vi "Write Page.vi"(4 "Additional Tags":T3(array[cluster]), 5 "Additional Named Tags":cluster{"name":string, "Variant":variant}[](array[cluster]), 6 "Settings":T4={"zlib compression level"=-1, "Max Strip bytes"=8192, "JPEG Quality (85)"=85}, 7 "Details":T5={"ImageDescription"="", "XResolution"=0.0, "YResolution"=0.0, "ResolutionUnit"=enum."Inch", "PhotometricInterpretation"=0, "Compression"=enum."None", "PageName"="", "DocumentName"=""} {"PhotometricInterpretation" items=["PHOTOMETRIC_MINISWHITE"=0, "PHOTOMETRIC_MINISBLACK"=1, "PHOTOMETRIC_RGB"=2, "PHOTOMETRIC_PALETTE"=3, "PHOTOMETRIC_MASK"=4, "PHOTOMETRIC_SEPARATED"=5, "PHOTOMETRIC_YCBCR"=6, "PHOTOMETRIC_CIELAB"=8, "PHOTOMETRIC_ICCLAB"=9, "PHOTOMETRIC_ITULAB"=10, "PHOTOMETRIC_LOGL"=32844, "PHOTOMETRIC_LOGLUV"=32845, "CFA"=32803, "LinearRaw"=34892, "DEPTH"=51177]}, 8 "error in (no error)":errorcluster, 10 "Image":variant, 11 "TIFF Writer in":refnum<class "TIFF Writer.lvclass">) -> (0 "error out":errorcluster, 3 "TIFF Writer out":refnum<class "TIFF Writer.lvclass">)   [LabVIEW 2020, in "LV Tiff.lvlib" / "TIFF Writer.lvclass"]
uses:
  TIFF Writer.lvclass
  _Helpers/Tiff Page Details.ctl
  _Helpers/Page Writer Settings.ctl
  _Helpers/Tiff Data Type.ctl
  TIFF Writer.lvclass/TIFF Writer.ctl
  _Helpers/Write IFD.vi
  LV Tiff.lvlib
  _Helpers/Tiff Tags.ctl
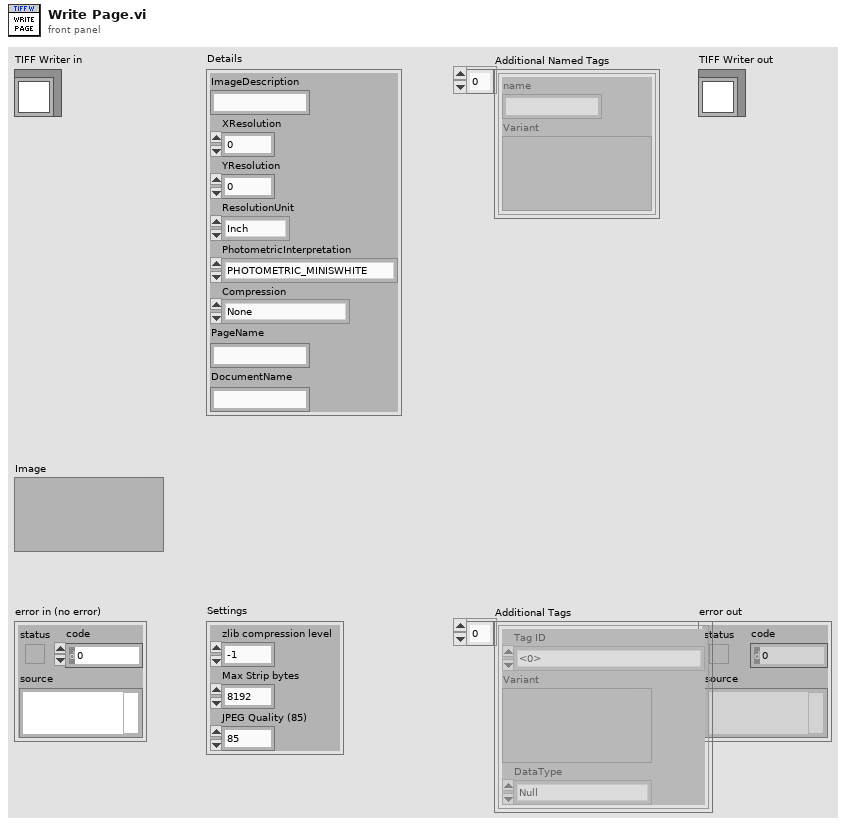
[diagram p1: front panel]
types:
  T1 = typedef "LV Tiff.lvlib/Tiff Tags.ctl" = u16
  T2 = typedef "LV Tiff.lvlib/Tiff Data Type.ctl" = enum16{"Null", "BYTE", "ASCII", "SHORT", "LONG", "RATIONAL", "SBYTE", "UNDEFINE", "SSHORT", "SLONG", "SRATIONAL", "FLOAT", "DOUBLE"}
  T3 = cluster{"Tag ID":T1, "Variant":variant, "DataType":T2}[]
  T4 = typedef "LV Tiff.lvlib/Page Writer Settings.ctl" = cluster{"zlib compression level":i32, "Max Strip bytes":u32, "JPEG Quality (85)":i32}
  T5 = typedef "LV Tiff.lvlib/Tiff Page Details.ctl" = cluster{"ImageDescription":string, "XResolution":dbl, "YResolution":dbl, "ResolutionUnit":enum16{"None", "Inch", "Centimeter"}, "PhotometricInterpretation":u16, "Compression":enum16{"None", "Deflate", "JPEG"}, "PageName":string, "DocumentName":string}
  T6 = enum16{"big-endian, network order", "native, host order", "little-endian"}
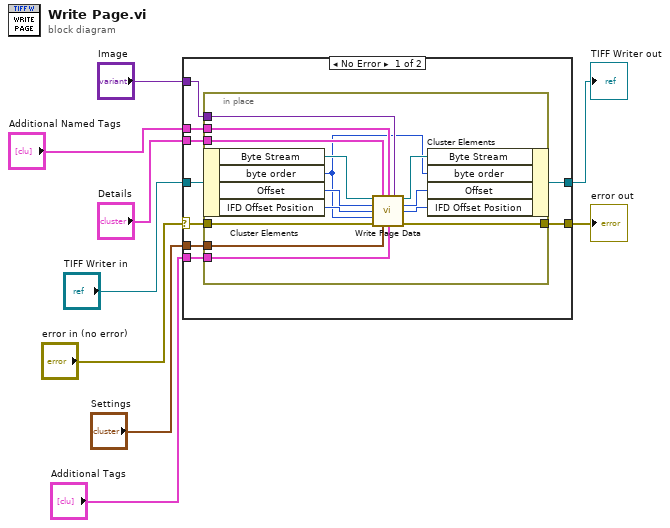
[diagram p0: block diagram]
diagram:
  n1 = case shown="No Error" "error in (no error)" {
    selector: "error in (no error)" -> [w16 w34]
    tunnel: [w15 w34] -> w8
    tunnel: [w17 w33] -> w6
    tunnel: "TIFF Writer in" -> [w18 w33]
    tunnel: "Additional Named Tags" -> [w14 _]
    tunnel: "Image" -> [w13 _]
    tunnel: "Details" -> [w12 _]
    tunnel: "Settings" -> [w11 _]
    tunnel: "Additional Tags" -> [w10 _]
    frame No Error {
      n2 = in-place {
        in-place-border: w16 -> [w32]
        in-place-border: [w31] -> w15
        in-place-border: w14 -> [w24]
        in-place-border: w13 -> [w23]
        in-place-border: w12 -> [w22]
        in-place-border: w11 -> [w20]
        in-place-border: w10 -> [w19]
        n3 = in-place-cluster #1(w18) -> ("Byte Stream"=w30:refnum<file>, "byte order"=w21:T6, "Offset"=w28:i32, "IFD Offset Position"=w27:i64)
        n4 = call "Write Page Data.vi"("Byte Stream File in"=w30, "Details"=w22, "Additional Named Tags"=w24, "Image"=w23, "Offset"=w28, "IFD Offset Position"=w27, "byte order (0:big-endian, network order)"=w21, "error in (no error)"=w32, "Settings"=w20, "Additional Tags"=w19) -> ("Byte Stream File out"=w29:refnum<file>, "Next Offset"=w26:i64, "Next IFD Offset Position"=w25:i64, "error out"=w31:errorcluster)  [unwired: 2 in]
        n5 = in-place-cluster #1("Byte Stream"=w29, "byte order"=w21, "Offset"=w26, "IFD Offset Position"=w25) -> (w17:refnum<class "TIFF Writer.lvclass">)
      }
    }
    frame Error {
    }
  }
  "error out" <- w8
  "TIFF Writer out" <- w6
